vi "2Slnd.vi"(8 "AllUp":bool, 9 "AllDown":bool, 10 "MostUp":bool, 11 "MostDown":bool) -> ()   [LabVIEW 2015]
uses:
  <vilib>/Rock Robotics/WPI/Solenoid/Deprecated/WPI_SolenoidSetBool.vi
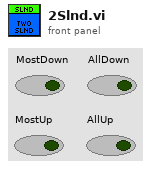
[diagram p1: front panel]
types:
  T1 = typedef "WPI_SolenoidDevRef.ctl" = cluster{"DevStatus":errorcluster, "Pneumatics Control Module":u8, "Forward Solenoid Channel":T2, "Reverse Solenoid Channel":T2}
  T2 = typedef "WPI_SolenoidChannel.ctl" = enum8{"Solenoid 0", "Solenoid 1", "Solenoid 2", "Solenoid 3", "Solenoid 4", "Solenoid 5", "Solenoid 6", "Solenoid 7", "Invalid"}
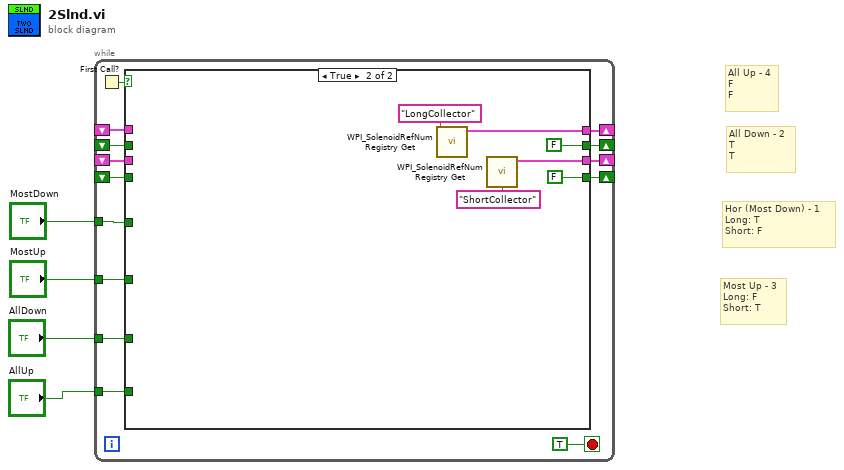
[diagram p0: block diagram]
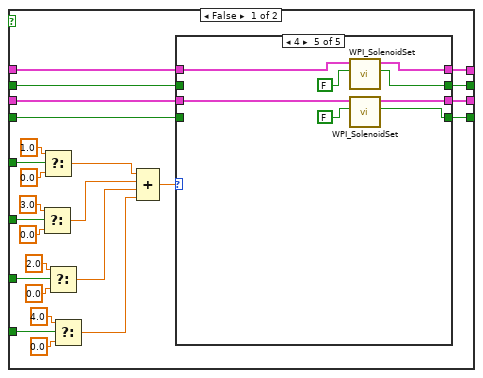
[diagram p2: hidden frame]
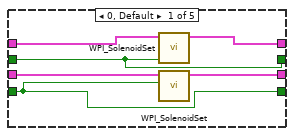
[diagram p3: hidden frame]
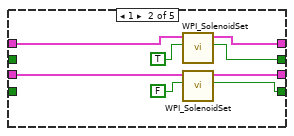
[diagram p4: hidden frame]
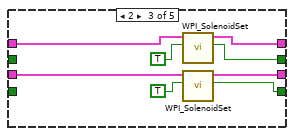
[diagram p5: hidden frame]
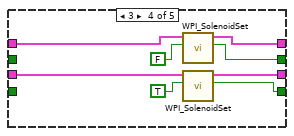
[diagram p6: hidden frame]
diagram:
  # "Most Up - 3\nLong: F\nShort: T"
  # "Hor (Most Down) - 1\nLong: T\nShort: F"
  # "All Down - 2\nT\nT"
  # "All Up - 4\nF\nF"
  n1 = while {
    shift-right: [w16] -> _
    shift-left: _ -> [w15]
    tunnel: "MostDown" -> [w14]
    shift-right: [w13] -> _
    shift-left: _ -> [w12]
    shift-right: [w11] -> _
    shift-left: _ -> [w5]
    shift-right: [w10] -> _
    shift-left: _ -> [w9]
    tunnel: "MostUp" -> [w8]
    tunnel: "AllDown" -> [w7]
    tunnel: "AllUp" -> [w6]
    stop <- TRUE stop-if-true
    n2 = First Call?() -> (First Call?: T/F=w17:bool)
    n3 = case shown="True" w17 {
      tunnel: [w25 w78] -> w16
      tunnel: w15 -> [w26 _]
      tunnel: w14 -> [w41 _]
      tunnel: [w23 FALSE] -> w13
      tunnel: w12 -> [w24 _]
      tunnel: [w21 w75] -> w11
      tunnel: [w19 FALSE] -> w10
      tunnel: w9 -> [w20 _]
      tunnel: w8 -> [w38 _]
      tunnel: w7 -> [w35 _]
      tunnel: w6 -> [w32 _]
      tunnel: w5 -> [w22 _]
      frame False {
        n4 = Select(t=3.0, s=w38, f=0.0 ("t")) -> (s? t:f=w29:dbl)
        n5 = Select(t=1.0, s=w41, f=0.0 ("t")) -> (s? t:f=w30:dbl)
        n6 = Select(t=2.0, s=w35, f=0.0 ("t")) -> (s? t:f=w28:dbl)
        n7 = Select(t=4.0, s=w32, f=0.0 ("t")) -> (s? t:f=w27:dbl)
        n8 = Compound Arithmetic op=ADD(w30, w29, w28, w27) -> (w31:dbl)
        n9 = case shown="4" w31 {
          tunnel: w26 -> [w47 w55 w61 w67 w73]
          tunnel: [w49 w54 w60 w66 w72] -> w25
          tunnel: w24 -> [w45 _ _ _ _]
          tunnel: [w45 w51 w57 w63 w69] -> w23
          tunnel: w22 -> [w46 w53 w59 w65 w71]
          tunnel: [w48 w52 w58 w64 w70] -> w21
          tunnel: w20 -> [w44 _ _ _ _]
          tunnel: [w44 w50 w56 w62 w68] -> w19
          frame 0, Default {
            n10 = call-poly <vilib>:"WPI_SolenoidSet.vi"("Value"=w45, "SolenoidDevRef"=w47) -> ("SolenoidDevRef"=w49:T1)  [unwired: 8 in, 1 out]
            n11 = call-poly <vilib>:"WPI_SolenoidSet.vi"("Value"=w44, "SolenoidDevRef"=w46) -> ("SolenoidDevRef"=w48:T1)  [unwired: 8 in, 1 out]
          }
          frame 1 {
            w50 = FALSE
            w51 = TRUE
            n12 = call-poly <vilib>:"WPI_SolenoidSet.vi"("Value"=w51, "SolenoidDevRef"=w55) -> ("SolenoidDevRef"=w54:T1)  [unwired: 8 in, 1 out]
            n13 = call-poly <vilib>:"WPI_SolenoidSet.vi"("Value"=w50, "SolenoidDevRef"=w53) -> ("SolenoidDevRef"=w52:T1)  [unwired: 8 in, 1 out]
          }
          frame 2 {
            w56 = TRUE
            w57 = TRUE
            n14 = call-poly <vilib>:"WPI_SolenoidSet.vi"("Value"=w57, "SolenoidDevRef"=w61) -> ("SolenoidDevRef"=w60:T1)  [unwired: 8 in, 1 out]
            n15 = call-poly <vilib>:"WPI_SolenoidSet.vi"("Value"=w56, "SolenoidDevRef"=w59) -> ("SolenoidDevRef"=w58:T1)  [unwired: 8 in, 1 out]
          }
          frame 3 {
            w62 = TRUE
            w63 = FALSE
            n16 = call-poly <vilib>:"WPI_SolenoidSet.vi"("Value"=w63, "SolenoidDevRef"=w67) -> ("SolenoidDevRef"=w66:T1)  [unwired: 8 in, 1 out]
            n17 = call-poly <vilib>:"WPI_SolenoidSet.vi"("Value"=w62, "SolenoidDevRef"=w65) -> ("SolenoidDevRef"=w64:T1)  [unwired: 8 in, 1 out]
          }
          frame 4 {
            w68 = FALSE
            w69 = FALSE
            n18 = call-poly <vilib>:"WPI_SolenoidSet.vi"("Value"=w69, "SolenoidDevRef"=w73) -> ("SolenoidDevRef"=w72:T1)  [unwired: 8 in, 1 out]
            n19 = call-poly <vilib>:"WPI_SolenoidSet.vi"("Value"=w68, "SolenoidDevRef"=w71) -> ("SolenoidDevRef"=w70:T1)  [unwired: 8 in, 1 out]
          }
        }
      }
      frame True {
        n20 = call <vilib>:"WPI_SolenoidRefNum Registry Get.vi"("refnum name"="LongCollector") -> ("SolenoidDevRef"=w78:T1)  [unwired: 9 in, 1 out]
        n21 = call <vilib>:"WPI_SolenoidRefNum Registry Get.vi"("refnum name"="ShortCollector") -> ("SolenoidDevRef"=w75:T1)  [unwired: 9 in, 1 out]
      }
    }
  }
